vi "PH_DIM.get Double.vi"(1 "no link":bool, 2 "typeDescriptor":string, 3 "data":i8[](array[numeric]), 4 "quality":i32) -> (0 "Value":dbl)   [LabVIEW 2014, in "PH_Common.lvlib"]
doc: "This VI calculates the status of double tag. It gives out:\n\n99999: no link or wrong data type or tag status bad\nelse: link and data type and tag status ok, value"
uses:
  PH_Common.lvlib
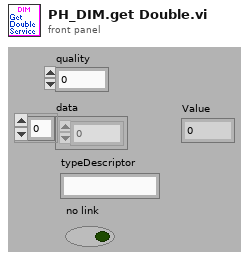
[diagram p1: front panel]
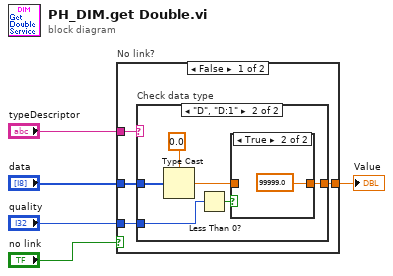
[diagram p0: block diagram]
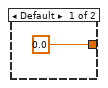
[diagram p2: hidden frame]
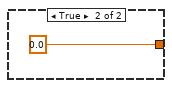
[diagram p4: hidden frame]
diagram:
  n1 = case "No link?" shown="False" "no link" {
    tunnel: [w9 0.0] -> w5
    tunnel: "quality" -> [w8 _]
    tunnel: "data" -> [w7 _]
    tunnel: "typeDescriptor" -> [w6 _]
    frame False {
      n2 = case "Check data type" shown="\"D\", \"D:1\"" w6 {
        tunnel: [0.0 w16] -> w9
        tunnel: w8 -> [_ w14]
        tunnel: w7 -> [_ w12]
        frame Default {
        }
        frame "D", "D:1" {
          n3 = Type Cast(type=0.0, x=w12) -> (*(type *) &x=w11:dbl)
          n4 = Less Than 0?(x=w14) -> (x < 0?=w15:bool)
          n5 = case shown="True" w15 {
            tunnel: [w17 99999.0] -> w16
            tunnel: w11 -> [w17 _]
            frame False {
            }
            frame True {
            }
          }
        }
      }
    }
    frame True {
    }
  }
  "Value" <- w5
